vi "E01_Tipo de datos.vi"() -> ()   [LabVIEW 2026]
panel:
  out "Array":dbl[](array[numeric])=[5.8]
  out "Cluster":cluster{"Numeric":dbl, "Numeric 2":dbl}
  out "String":string
  out "Numeric 4":i32=5
  out "Numeric 3":dbl=5.3
  out "Numeric 2":i32
  out "Numeric":dbl
  out "Tank":dbl(slide) scale=0.0..10.0
  in  "Entero":i32
  in  "Doble":dbl
  in  "Contol":bool
  out "Led_03":bool
  out "Led_02":bool
  out "Led_01":bool
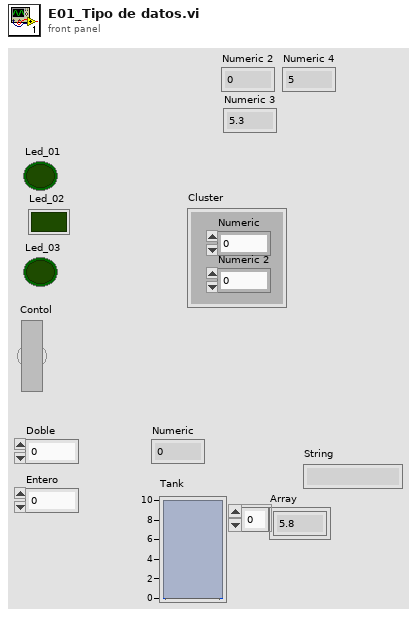
[diagram p1: front panel]
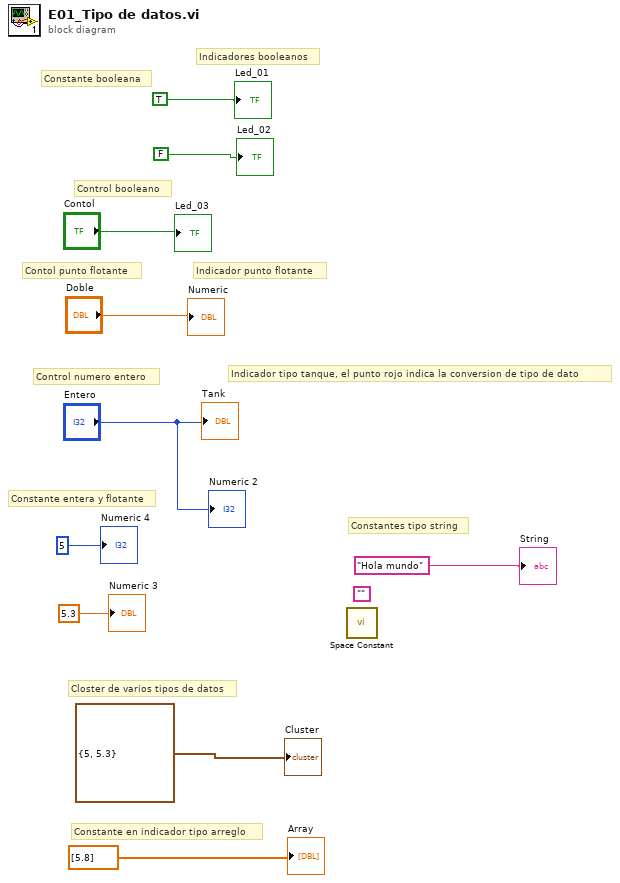
[diagram p0: block diagram]
diagram:
  (unwired) ""
  # "Constante en indicador tipo arreglo"
  # "Closter de varios tipos de datos"
  # "Constante entera y flotante"
  # "Constantes tipo string"
  # "Indicador tipo tanque, el punto rojo indica la conversion de tipo de dato"
  # "Indicador punto flotante"
  # "Control numero entero"
  # "Contol punto flotante"
  # "Control booleano"
  # "Indicadores booleanos"
  # "Constante booleana"
  n1 = call <vilib>:"Space Constant.vi"() -> ()  [unwired: 1 out]
  "Led_01" <- TRUE
  "Led_02" <- FALSE
  "Led_03" <- "Contol"
  "Tank" <- "Entero"
  "Numeric" <- "Doble"
  "Numeric 2" <- "Entero"
  "Numeric 3" <- 5.3
  "Numeric 4" <- 5
  "String" <- "Hola mundo"
  "Cluster" <- cluster{i32, dbl} {5, 5.3}
  "Array" <- dbl[] [5.8]
